vi "Cfg List _ Get Current Configurations.vi"(6 "ColInfo.ColName[]":string[](array[string]), 8 "error in":errorcluster caption="错误输入", 11 "tree":refnum<vi>) -> (0 "error out":errorcluster caption="错误输出", 2 "TreePara":cluster{"ColHdrs":string[], "Items":string[][]})   [LabVIEW 2016]
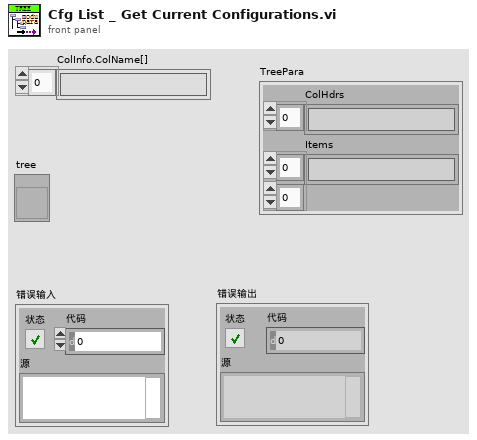
[diagram p1: front panel]
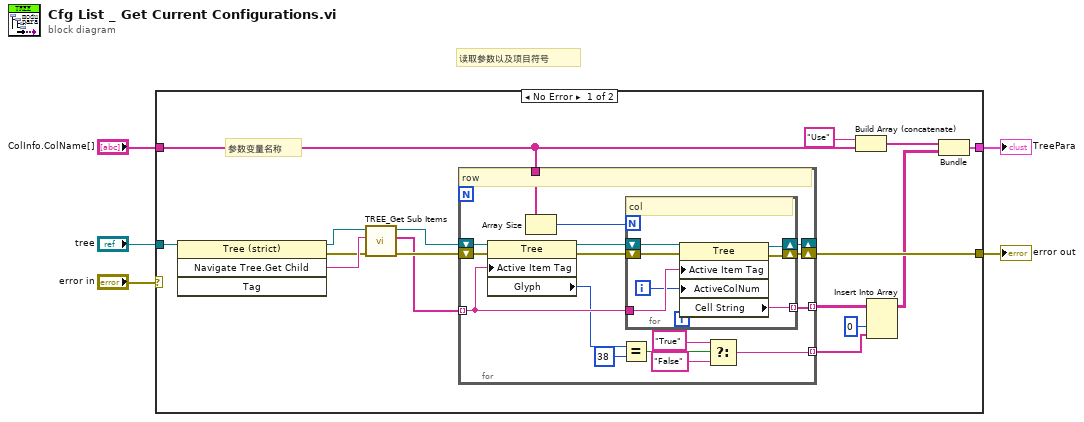
[diagram p0: block diagram]
diagram:
  # "读取参数以及项目符号"
  n1 = case shown="No Error" "error in" {
    selector: "error in" -> [_ w45]
    tunnel: [w15 w45] -> w4
    tunnel: "tree" -> [w21 _]
    tunnel: "ColInfo.ColName[]" -> [w10 _]
    tunnel: [w6 _] -> w1
    frame No Error {
      # "参数变量名称"
      n2 = invoke class="Tree (strict)" method="Navigate Tree.Get Child"(reference=w21) -> (reference out=w20:refnum<vi>, error out=w18:errorcluster, "Navigate Tree:Get Child"=w19:string)  [unwired: 3 in, 1 out]
      n3 = call "TREE_Get Sub Items.vi"("error in"=w18, "Par Tag"=w19, "TreeRef"=w20) -> ("error out"=w16:errorcluster, "Tags"=w9:string[], "TreeRef"=w17:refnum<vi>)  [unwired: 5 in, 1 out]
      n4 = for {
        tunnel: w9 -> [w28] mode=indexing
        shift-right: [w35] -> _
        shift-left: w17 -> [w32]
        tunnel: [w37] -> w13 mode=indexing
        shift-right: [w36] -> w15
        shift-left: w16 -> [w31]
        tunnel: w10 -> [w34]
        tunnel: [w22] -> w11 mode=indexing
        # "row"
        n5 = property class="Tree"(reference=w32, error in=w31, "Active Item Tag"=w28) -> (reference out=w30:refnum<vi>, error out=w29:errorcluster, "Glyph"=w26:i32)
        n6 = Array Size(array=w34) -> (size(s)=w33:i32)
        n7 = Equal?(x=w26, y=38) -> (x = y?=w27:bool)
        n8 = for {
          N: w33 -> [_]
          tunnel: w28 -> [w44]
          tunnel: [w40] -> w37 mode=indexing
          shift-right: [w39] -> w36
          shift-left: w29 -> [w42]
          shift-right: [w38] -> w35
          shift-left: w30 -> [w43]
          i -> [w41]
          # "col"
          n9 = property class="Tree"(reference=w43, error in=w42, "Active Item Tag"=w44, "ActiveColNum"=w41) -> (reference out=w38:refnum<vi>, error out=w39:errorcluster, "Cell String"=w40:string)
        }
        n10 = Select(t="True", s=w27, f="False") -> (s? t:f=w22:string)
      }
      n11 = Build Array (concatenate)("Use", w10) -> (w8:string[])
      n12 = Insert Into Array(array=w13, index (col)=0 ("禁用的索引 (列)"), new element=w11) -> (w7:string[][])  [unwired: 1 in]
      n13 = Bundle(w8, w7) -> (w6:cluster{string[], string[][]})  [unwired: 1 in]
    }
    frame Error {
    }
  }
  "error out" <- w4
  "TreePara" <- w1
